vi "InspectTellCleanup.vi"(6 "Error":errorcluster, 7 "Actor":refnum<class "Actor Layer.lvclass">, 10 "Msg":T1 {"Msg Attribs"."Listen Absolute Time" format="%<%x %.3X>T"; "Msg Attribs"."Tell Absolute Time" format="%<%x %.3X>T"}, 11 "Actor":T5) -> (2 "Msg":T1 {"Msg Attribs"."Listen Absolute Time" format="%<%x %.3X>T"; "Msg Attribs"."Tell Absolute Time" format="%<%x %.3X>T"}, 3 "Actor":T5, 4 "Error":errorcluster, 5 "Actor":refnum<class "Actor Layer.lvclass">)   [LabVIEW 2020, in "_Template.lvlib" / "{{Actor}}.lvlib" / "Actor Layer.lvclass"]
uses:
  Actor Layer.lvclass
  Actor Layer.lvclass/Actor Layer.ctl
  jettl/jettl/Actor Layer/Actor Layer.lvclass
  jettl/jettl/Msg/Msg.lvclass
  jettl/jettl/Origin.ctl
  jettl/jettl/jettl.lvlib
  jettl/jettl/Lifecycle.ctl
  jettl/jettl/Msg Attribs.ctl
  jettl/jettl/Msg.ctl
  jettl/jettl/Post Setup.ctl
  jettl/jettl/Pre Setup.ctl
  jettl/jettl/Msg Set.ctl
  jettl/jettl/Actor Attribs.ctl
  jettl/jettl/Children.ctl
  jettl/jettl/Actor.ctl
  jettl/jettl/Layer Type.ctl
  jettl/jettl/Layer Attribs.ctl
  jettl/jettl/Layer Map.ctl
  jettl/jettl/Implemented Map.ctl
panel:
  # "This front panel should not be manipulated."
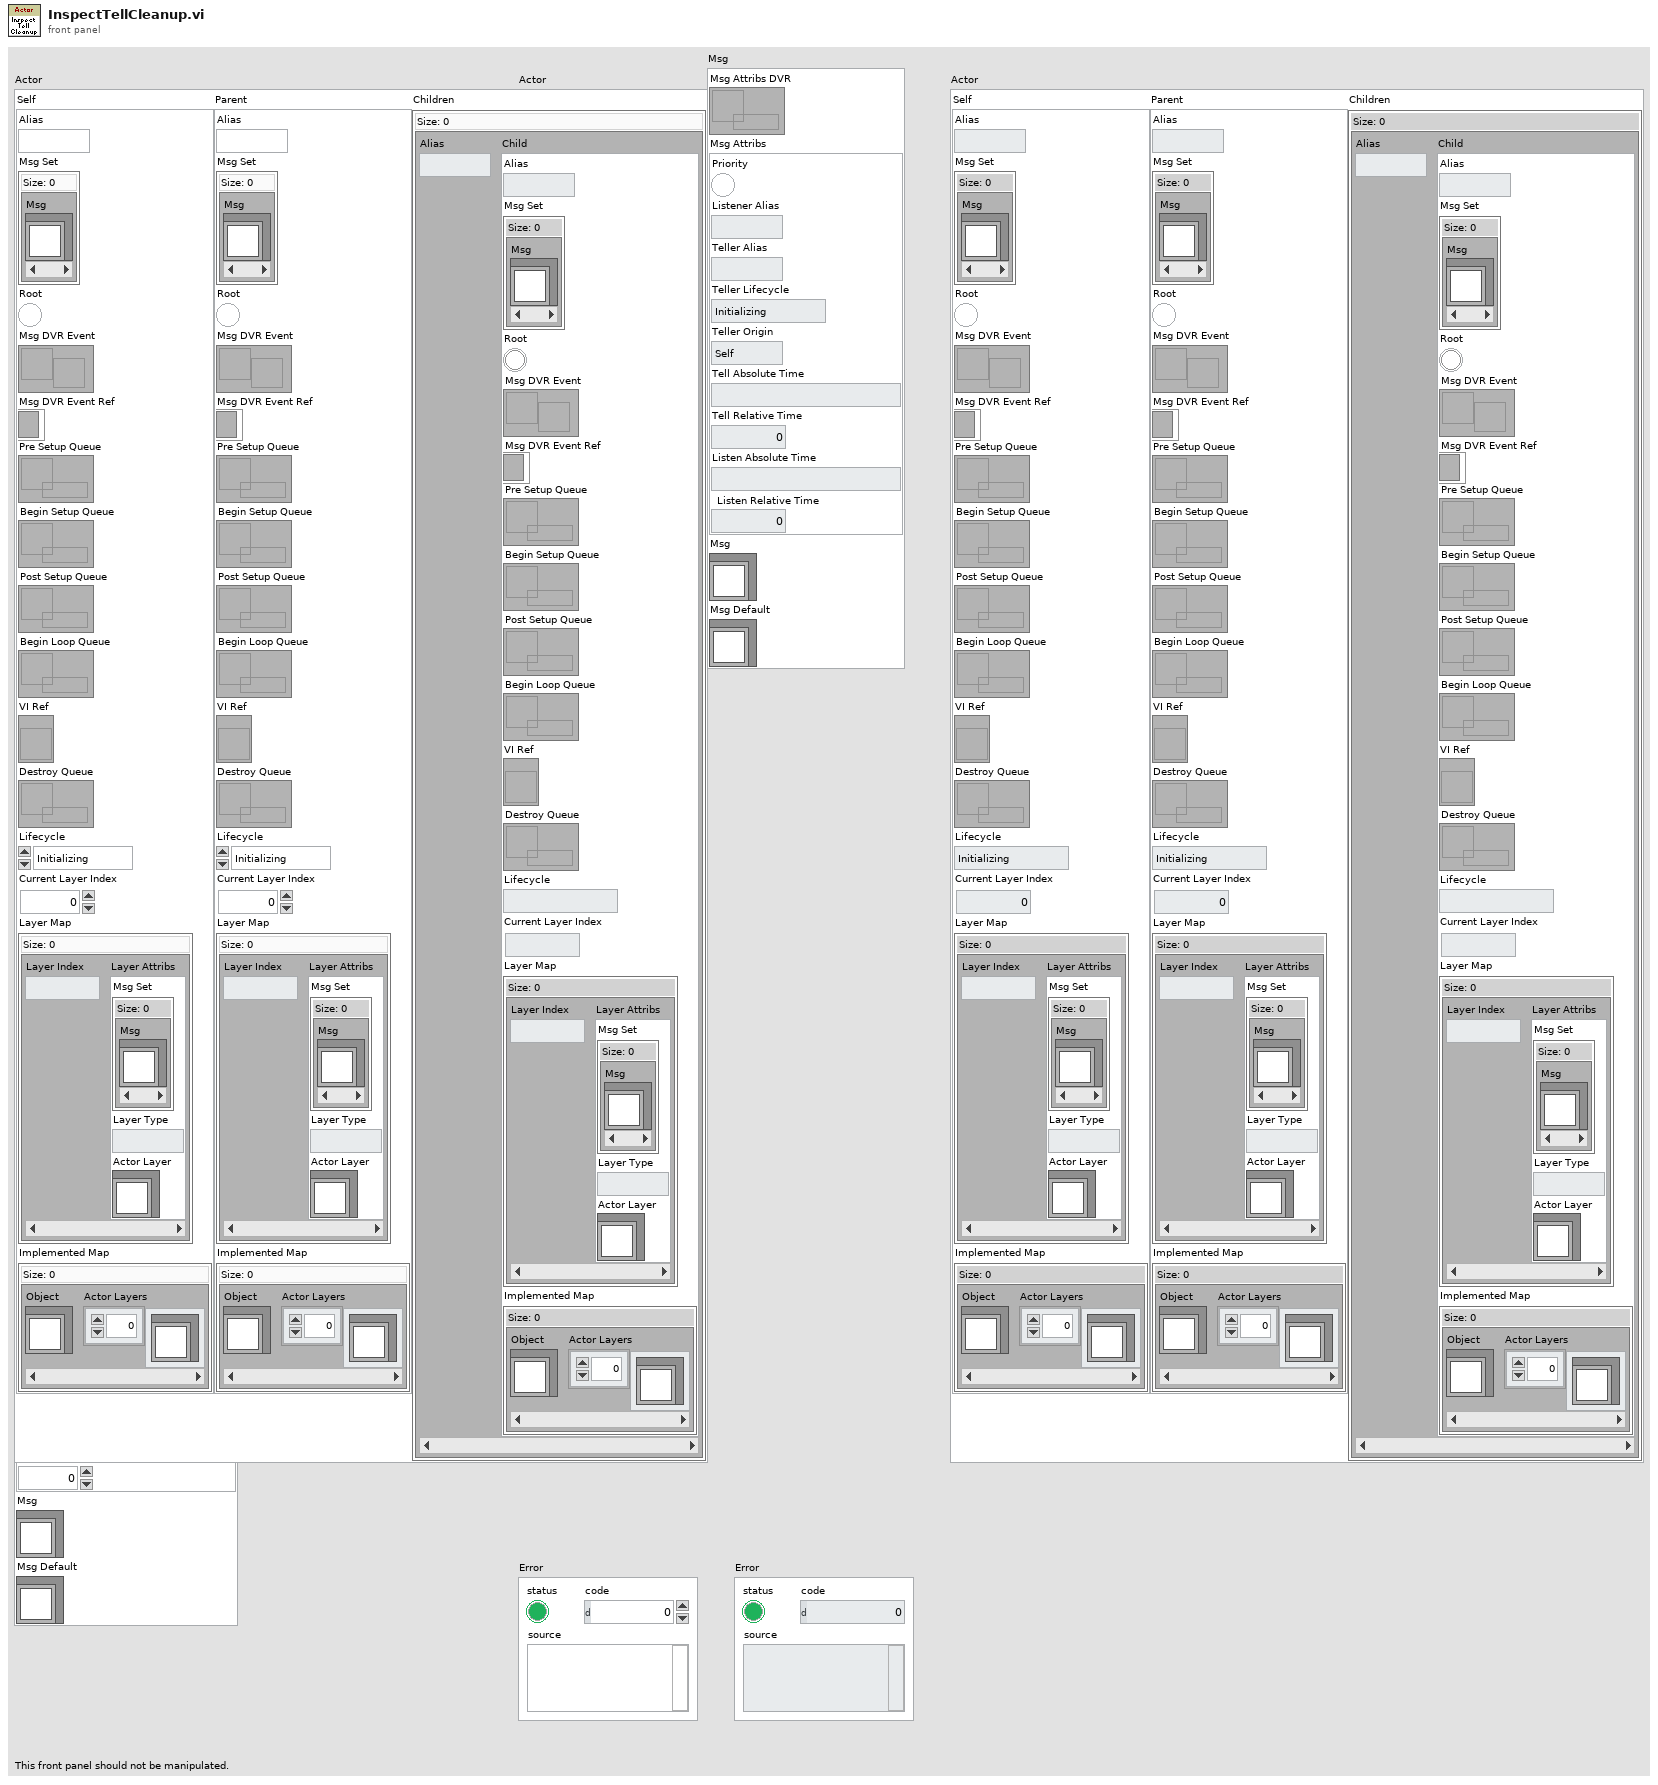
[diagram p1: front panel]
types:
  T1 = typedef "jettl.lvlib/Msg.ctl" = cluster{"Msg Attribs DVR":refnum<data-value>, "Msg Attribs":T2, "Msg":refnum<class "Msg.lvclass">, "Msg Default":refnum<class "Msg.lvclass">}
  T2 = typedef "jettl.lvlib/Msg Attribs.ctl" = cluster{"Priority":bool, "Listener Alias":string, "Teller Alias":string, "Teller Lifecycle":T3, "Teller Origin":T4, "Tell Absolute Time":timestamp, "Tell Relative Time":dbl, "Listen Absolute Time":timestamp, "Listen Relative Time":dbl}
  T3 = typedef "jettl.lvlib/Lifecycle.ctl" = enum16{"Initializing", "Setting Up", "Starting", "Running", "Stopping", "Tearing Down", "Terminated"}
  T4 = typedef "jettl.lvlib/Origin.ctl" = enum16{"Self", "Parent", "Child"}
  T5 = typedef "jettl.lvlib/Actor.ctl" = cluster{"Self":T6, "Parent":T6, "Children":T12}
  T6 = typedef "jettl.lvlib/Actor Attribs.ctl" = cluster{"Alias":string, "Msg Set":T7, "Root":bool, "Msg DVR Event":refnum<user-event>, "Msg DVR Event Ref":refnum<event-registration>, "Pre Setup Queue":refnum<queue>, "Begin Setup Queue":refnum<queue>, "Post Setup Queue":refnum<queue>, "Begin Loop Queue":refnum<queue>, "VI Ref":refnum<vi>, "Destroy Queue":refnum<queue>, "Lifecycle":T3, "Current Layer Index":i32, "Layer Map":T8, "Implemented Map":T11}
  T7 = typedef "jettl.lvlib/Msg Set.ctl" = set{refnum<class "Msg.lvclass">}
  T8 = typedef "jettl.lvlib/Layer Map.ctl" = map{i32, T9}
  T9 = typedef "jettl.lvlib/Layer Attribs.ctl" = cluster{"Msg Set":T7, "Layer Type":T10, "Actor Layer":refnum<class "Actor Layer.lvclass">}
  T10 = typedef "jettl.lvlib/Layer Type.ctl" = enum16{"Base", "InnerGlobal", "InnerLocal", "Outer"}
  T11 = typedef "jettl.lvlib/Implemented Map.ctl" = map{refnum<class>, refnum<class "Actor Layer.lvclass">[]}
  T12 = typedef "jettl.lvlib/Children.ctl" = map{string, T6}
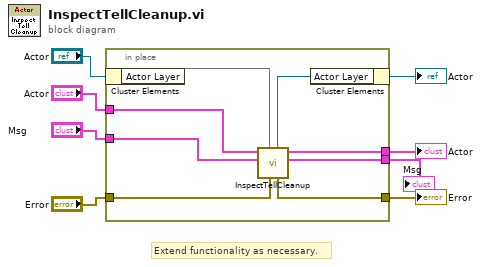
[diagram p0: block diagram]
diagram:
  # "Extend functionality as necessary."
  n1 = in-place {
    in-place-border: "Msg" -> [w12]
    in-place-border: "Error" -> [w14]
    in-place-border: [w13] -> w4
    in-place-border: "Actor" -> [w11]
    in-place-border: [w10] -> w2
    in-place-border: [w9] -> w1
    n2 = in-place-cluster #1("Actor") -> ("Actor Layer"=w16)
    n3 = call-dynamic "InspectTellCleanup.vi"("Error"=w14, 7:"Actor"=w16, "Msg"=w12, 11:"Actor"=w11) -> ("Msg"=w9:T1, 3:"Actor"=w10:T5, "Error"=w13:errorcluster, 5:"Actor"=w15:refnum<class "Actor Layer.lvclass">)  [unwired: 4 in]
    n4 = in-place-cluster #1("Actor Layer"=w15) -> (→"Actor":refnum<class "Actor Layer.lvclass">)
  }
  "Error" <- w4
  "Actor" <- w2
  "Msg" <- w1
